vi "Tiff saver.vi"(7 "Status":T1 {"Setting"."X Pos." scale=-2.0..2.0; "Setting"."Y Pos." scale=-2.0..2.0}, 8 "error in (no error)":errorcluster, 10 "File Path":path, 11 "Image in":T4) -> (0 "error out":errorcluster)   [LabVIEW 2013]
uses:
  Image.ctl
  init & communication/init-status.ctl
  init & communication/Setting.ctl
  init & communication/event-package.ctl
  init & communication/Event1.ctl
  init & communication/data-package.ctl
  init & communication/Event.ctl
panel:
  out "无符号16位整型":u16[][](array[numeric])
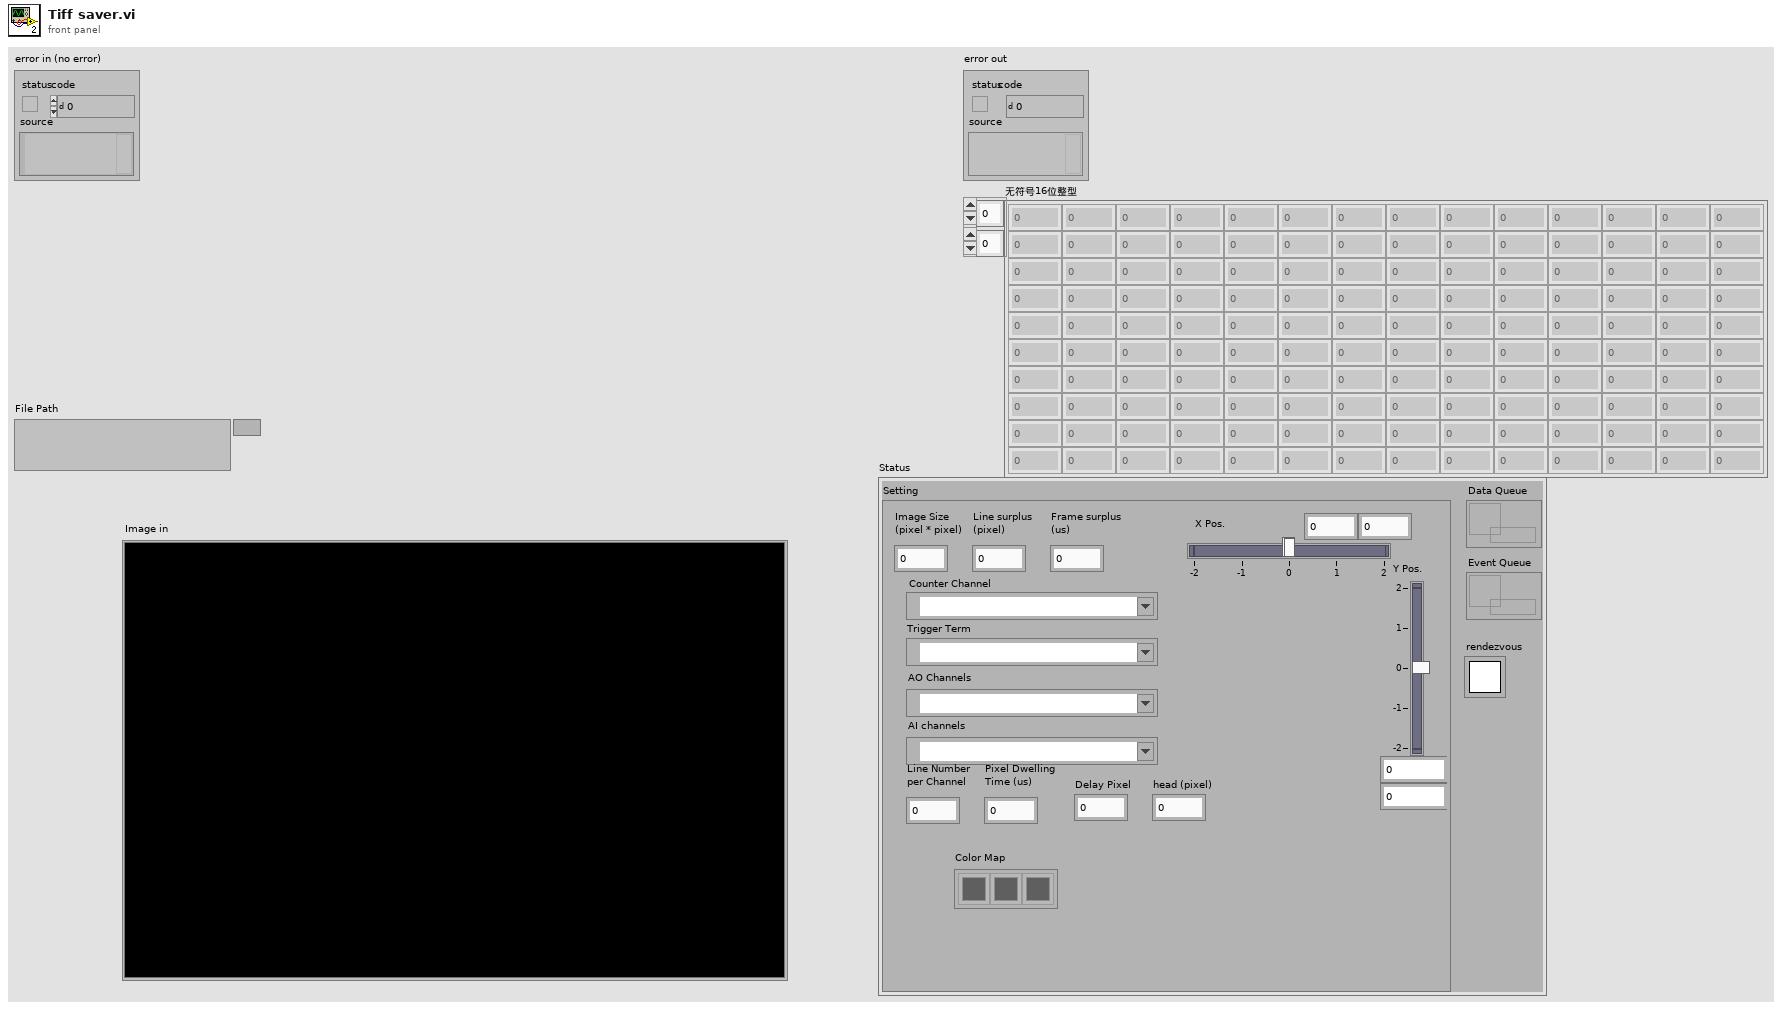
[diagram p1: front panel]
types:
  T1 = typedef "init-status.ctl" = cluster{"Setting":T2, "Event Queue":refnum<queue>, "Data Queue":refnum<queue>, "rendezvous":T3}
  T2 = typedef "Setting.ctl" = cluster{"Image Size\n(pixel * pixel)":i32, "Counter Channel":tag, "Trigger Term":tag, "AO Channels":tag, "Y Pos.":cluster{dbl, dbl}, "X Pos.":cluster{dbl, dbl}, "Line surplus\n(pixel)":i32, "Frame surplus\n(us)":i32, "AI channels":tag, "Line Number\nper Channel":i32, "Delay Pixel":i32, "Pixel Dwelling\nTime (us)":i32, "Color Map":u32[], "head (pixel)":i32}
  T3 = typedef "Rendezvous RefNum" = refnum<k1>
  T4 = typedef "Image.ctl" = dbl[][]
  T5 = typedef "Image Type" = u32
  T6 = typedef "IMAQ Image.ctl" = refnum<image>
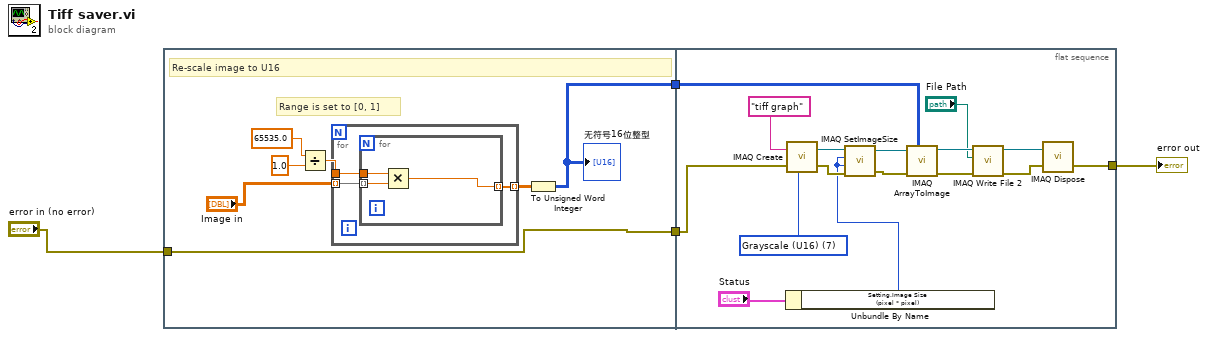
[diagram p0: block diagram]
diagram:
  n1 = flat-sequence {
    tunnel: [w10] -> w4
    tunnel: [w9] -> w2
    tunnel: "error in (no error)" -> [w9]
    tunnel: w4 -> [w18]
    tunnel: [w20] -> w3
    tunnel: w2 -> [w19]
    frame #0 {
      # "Range is set to [0, 1]"
      # "Re-scale image to U16"
      n2 = Divide(x=65535.0, y=1.0) -> (x/y=w6:dbl)
      n3 = for {
        tunnel: "Image in" -> [w14] mode=indexing
        tunnel: [w13] -> w11 mode=indexing
        tunnel: w6 -> [w12]
        n4 = for {
          tunnel: [w16] -> w13 mode=indexing
          tunnel: w14 -> [w17] mode=indexing
          tunnel: w12 -> [w15]
          n5 = Multiply(x=w15, y=w17) -> (x*y=w16:dbl)
        }
      }
      n6 = To Unsigned Word Integer(number=w11) -> (unsigned 16bit integer=w10:u16[][])
      "无符号16位整型" <- w10
    }
    frame #1 {
      w23 = T5 7 items=["Grayscale (U8)", "Grayscale (I16)", "Grayscale (SGL)", "Complex (CSG)", "RGB (U32)", "HSL (U32)", "RGB (U64)", "Grayscale (U16)"] ("Image Type")
      n7 = Unbundle By Name("Status") -> ("Setting.Image Size\n(pixel * pixel)"=w21:i32)
      n8 = call "IMAQ Create"("Image Name"="tiff graph", "Image Type"=w23, "error in (no error)"=w19) -> ("New Image"=w30:T6, "error out"=w31:errorcluster)  [unwired: 2 in]
      n9 = call "IMAQ SetImageSize"("error in (no error)"=w31, "Y Resolution"=w21, "X Resolution"=w21, "Image"=w30) -> ("error out"=w33:errorcluster, "Image Out"=w32:T6)  [unwired: 1 in]
      n10 = call "IMAQ ArrayToImage"("Image Pixels (U16)"=w18, "error in (no error)"=w33, "Image"=w32) -> ("error out"=w25:errorcluster, "Image Out"=w28:T6)  [unwired: 7 in]
      n11 = call-poly "IMAQ Write File 2"("error in (no error)"=w25, "File Path"="File Path", "Image"=w28) -> ("error out"=w26:errorcluster, "Image Out (duplicate)"=w27:T6)  [unwired: 7 in]
      n12 = call "IMAQ Dispose"("Image"=w27, "error in (no error)"=w26) -> ("error out"=w20:errorcluster)  [unwired: 4 in]
    }
  }
  "error out" <- w3
